vi "TestMALO(mismoVI).vi"() -> ()   [LabVIEW 2010]
panel:
  in  "Mensajes":T1(ring)
  in  "stop":bool
  in  "Send":bool=TRUE
  out "error out":errorcluster
  out "Respuesta":string
  out "Mensaje":string
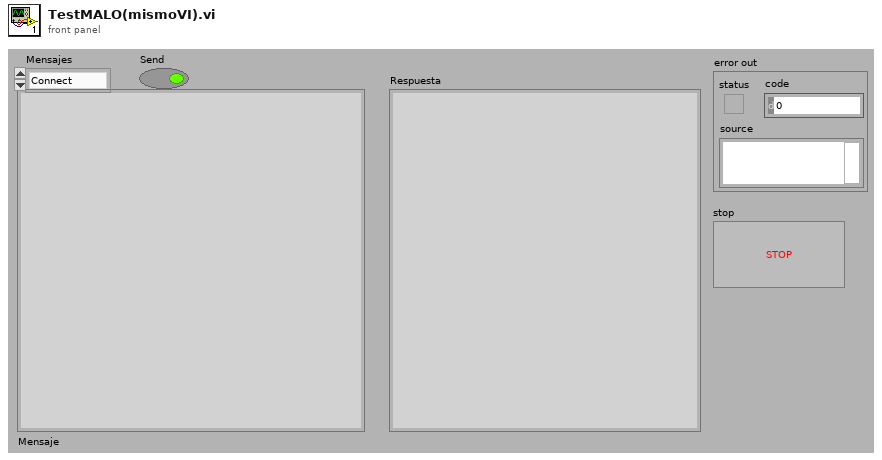
[diagram p1: front panel]
types:
  T1 = enum16{"Connect", "OpenVi", "RunVi", "StopVi", "CloseVi", "Disconnect"}
  T2 = enum16{"Standard", "Buffered", "CRLF", "Immediate"}
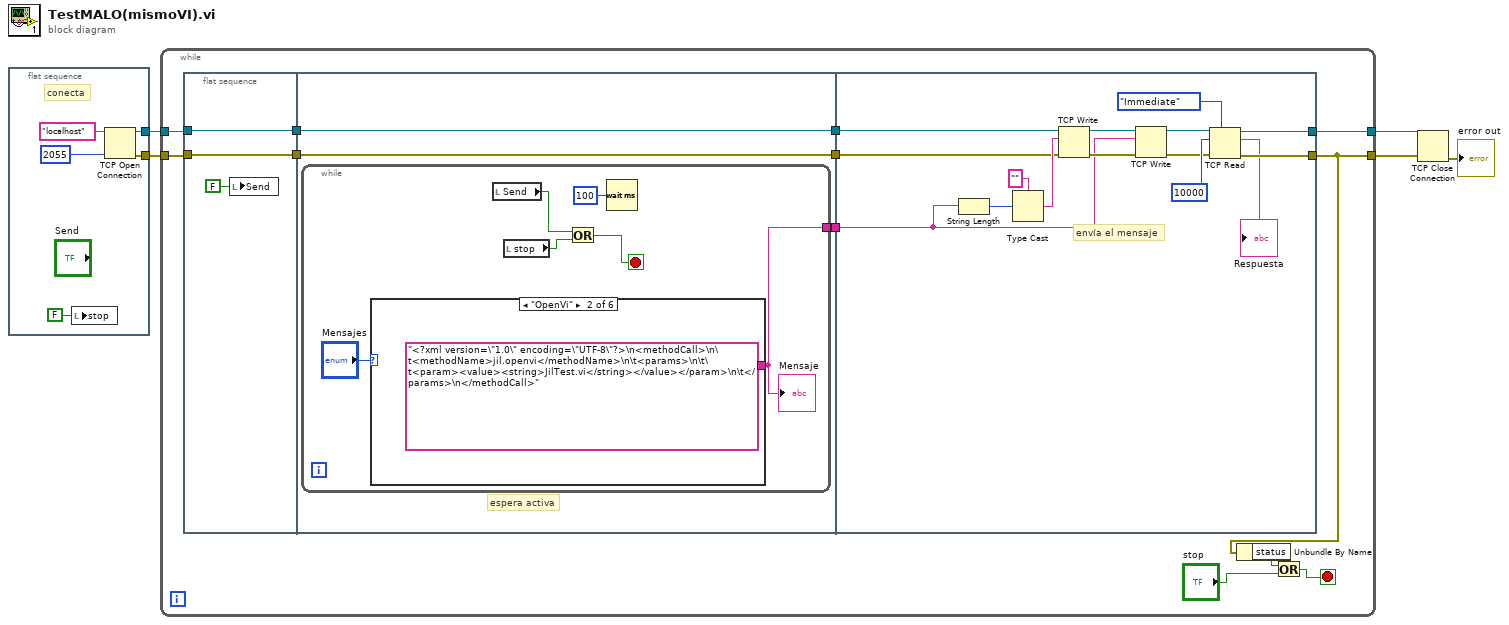
[diagram p0: block diagram]
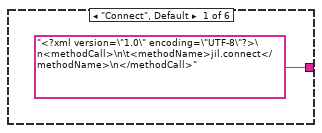
[diagram p2: hidden frame]
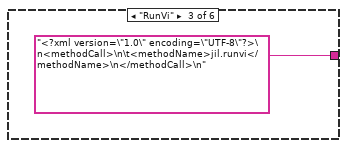
[diagram p3: hidden frame]
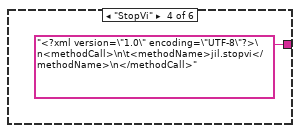
[diagram p4: hidden frame]
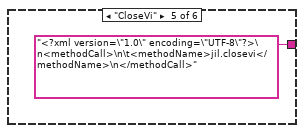
[diagram p5: hidden frame]
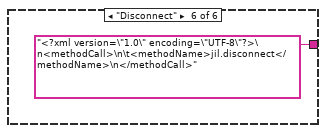
[diagram p6: hidden frame]
diagram:
  n1 = flat-sequence {
    tunnel: [w8] -> w5
    tunnel: [w7] -> w4
    frame #0 {
      # "conecta"
      n2 = local write "stop"(FALSE ("stop")) -> ()
      n3 = TCP Open Connection(address="localhost", remote port or service name=u16 2055) -> (connection ID=w8:refnum<k5>, error out=w7:errorcluster)  [unwired: 3 in]
    }
  }
  n4 = while {
    tunnel: w5 -> [w18]
    tunnel: w4 -> [w17]
    tunnel: [w16] -> w2
    tunnel: [w13] -> w1
    stop <- w14 stop-if-true
    n5 = flat-sequence {
      tunnel: w17 -> [w24]
      tunnel: [w24] -> w22
      tunnel: w18 -> [w23]
      tunnel: [w23] -> w21
      tunnel: w22 -> [w28]
      tunnel: [w28] -> w20
      tunnel: w21 -> [w27]
      tunnel: [w27] -> w19
      tunnel: [w26] -> w11
      tunnel: [w46] -> w16
      tunnel: [w45] -> w13
      tunnel: w20 -> [w44]
      tunnel: w19 -> [w43]
      tunnel: w11 -> [w41]
      frame #0 {
        n6 = local write "Send"(FALSE ("Send")) -> ()
      }
      frame #1 {
        # "espera activa"
        n7 = while {
          tunnel: [w29] -> w26
          stop <- w33 stop-if-true
          n8 = case shown="\"OpenVi\"" "Mensajes" {
            tunnel: ["<?xml version=\"1.0\" encoding=\"UTF-8\"?>\n<methodCall>\n\t<methodName>jil.connect</methodName>\n</methodCall>" "<?xml version=\"1.0\" encoding=\"UTF-8\"?>\n<methodCall>\n\t<methodName>jil.openvi</methodName>\n\t<params>\n\t\t<param><value><string>JilTest.vi</string></value></param>\n\t</params>\n</methodCall>" "<?xml version=\"1.0\" encoding=\"UTF-8\"?>\n<methodCall>\n\t<methodName>jil.runvi</methodName>\n</methodCall>\n" "<?xml version=\"1.0\" encoding=\"UTF-8\"?>\n<methodCall>\n\t<methodName>jil.stopvi</methodName>\n</methodCall>" "<?xml version=\"1.0\" encoding=\"UTF-8\"?>\n<methodCall>\n\t<methodName>jil.closevi</methodName>\n</methodCall>" "<?xml version=\"1.0\" encoding=\"UTF-8\"?>\n<methodCall>\n\t<methodName>jil.disconnect</methodName>\n</methodCall>"] -> w29
            frame "Connect", Default {
            }
            frame "OpenVi" {
            }
            frame "RunVi" {
            }
            frame "StopVi" {
            }
            frame "CloseVi" {
            }
            frame "Disconnect" {
            }
          }
          "Mensaje" <- w29
          n9 = local read "Send"() -> (w31:bool)
          n10 = local read "stop"() -> (w32:bool)
          n11 = Or(x=w31, y=w32) -> (x .or. y?=w33:bool)
          n12 = Wait (ms)(milliseconds to wait=u32 100) -> ()  [unwired: 1 out]
        }
      }
      frame #2 {
        # "envía el mensaje"
        n13 = String Length(string=w41) -> (length=w49:i32)
        n14 = Type Cast(type="", x=w49) -> (*(type *) &x=w51:string)
        n15 = TCP Write(connection ID=w43, data in=w51, error in (no error)=w44) -> (connection ID out=w47:refnum<k5>, error out=w48:errorcluster)  [unwired: 1 in, 1 out]
        n16 = TCP Write(connection ID=w47, data in=w41, error in (no error)=w48) -> (connection ID out=w52:refnum<k5>, error out=w53:errorcluster)  [unwired: 1 in, 1 out]
        n17 = TCP Read(connection ID=w52, bytes to read=10000, error in (no error)=w53, 7:T2."Immediate" ("mode (standard)")) -> (connection ID out=w46:refnum<k5>, data out=→"Respuesta":string, error out=w45:errorcluster)  [unwired: 1 in]
      }
    }
    n18 = Unbundle By Name(w13) -> ("status"=w12:bool)
    n19 = Or(x=w12, y="stop") -> (x .or. y?=w14:bool)
  }
  n20 = TCP Close Connection(connection ID=w2, error in (no error)=w1) -> (error out=→"error out":errorcluster)  [unwired: 1 in, 1 out]
